vi "ep_EN50160 Basic Statistical Evaluation (1D).vi"(0 "data":dbl[](array[numeric]), 1 "evaluated data":enum16{"all data", "data without flag"}(ring), 5 "data flags":bool[](array[boolean]), 7 "EN50160 limits":T2={"upper limit"=110.0, "lower limit"=90.0, "required percentage to be in limits"=95.0}, 11 "error in (no error)":errorcluster) -> (4 "EN50160 result":T1, 10 "passed?":bool, 15 "error out":errorcluster)   [LabVIEW 2011, in "NI_EP_Power Quality.lvlib"]
uses:
  <vilib>/addons/Electrical Power/PQ/NI_EP_Power Quality.lvlib
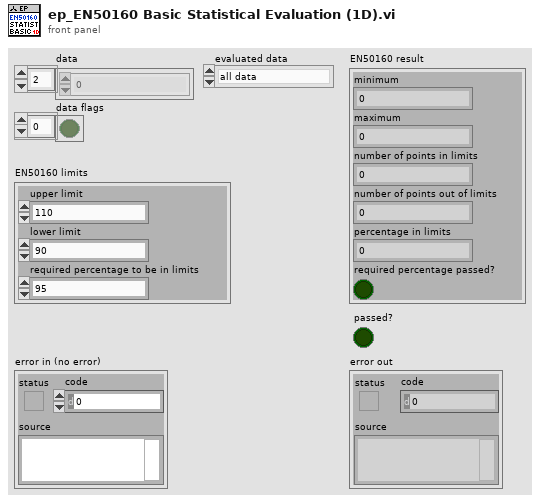
[diagram p1: front panel]
types:
  T1 = cluster{"minimum":dbl, "maximum":dbl, "number of points in limits":u32, "number of points out of limits":u32, "percentage in limits":dbl, "required percentage passed?":bool}
  T2 = cluster{"upper limit":dbl, "lower limit":dbl, "required percentage to be in limits":dbl}
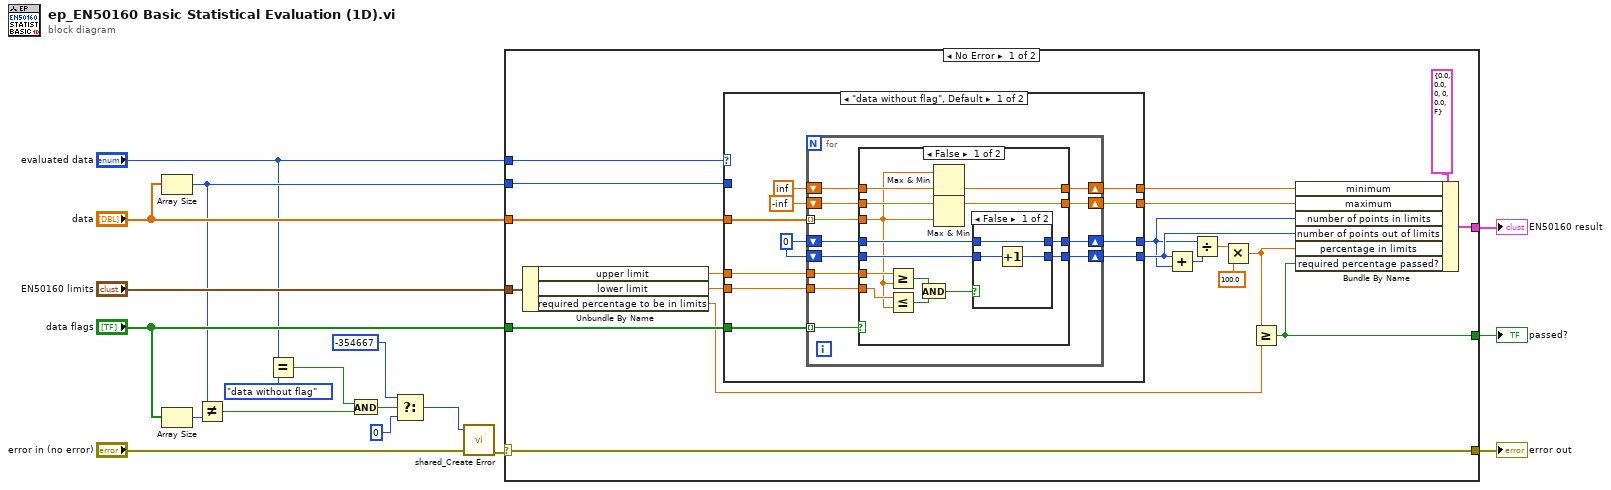
[diagram p0: block diagram]
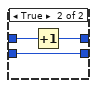
[diagram p2: hidden frame]
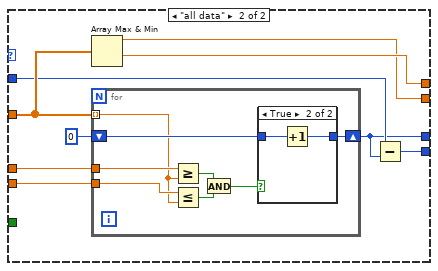
[diagram p4: hidden frame]
diagram:
  n1 = Array Size(array="data") -> (size(s)=w12:i32)
  n2 = Array Size(array="data flags") -> (size(s)=w16:i32)
  n3 = Not Equal?(x=w12, y=w16) -> (x != y?=w11:bool)
  n4 = Equal?(x="evaluated data", y=enum16{"all data", "data without flag"}."data without flag") -> (x = y?=w7:bool)
  n5 = And(x=w7, y=w11) -> (x .and. y?=w10:bool)
  n6 = Select(t=-354667 ("error code (0)"), s=w10, f=0 ("error code (0)")) -> (s? t:f=w1:i32)
  n7 = call <vilib>:"shared_Create Error.vi"("error in (no error)"="error in (no error)", "error code (0)"=w1) -> ("error out"=w2:errorcluster)  [unwired: 9 in]
  n8 = case shown="No Error" w2 {
    selector: w2 -> [w35 w106]
    tunnel: "evaluated data" -> [w33 _]
    tunnel: "data" -> [w34 _]
    tunnel: "data flags" -> [w38 _]
    tunnel: [w35 w106] -> w15
    tunnel: [w36 _] -> w14
    tunnel: "EN50160 limits" -> [w32 _]
    tunnel: w12 -> [w21 _]
    tunnel: [w19 _] -> w6
    frame No Error {
      n9 = Unbundle By Name(w32) -> ("upper limit"=w31:dbl, "lower limit"=w30:dbl, "required percentage to be in limits"=w22:dbl)
      n10 = case shown="\"data without flag\", Default" w33 {
        tunnel: w38 -> [w45 _]
        tunnel: w30 -> [w43 w92]
        tunnel: w34 -> [w49 w91]
        tunnel: w31 -> [w44 w93]
        tunnel: [w42 w90] -> w29
        tunnel: [w41 w89] -> w28
        tunnel: [w40 w87] -> w20
        tunnel: [w39 w86] -> w27
        tunnel: w21 -> [_ w88]
        frame "data without flag", Default {
          w48 = u32 0 ("number of points in limits")
          n11 = for {
            tunnel: w49 -> [w56] mode=indexing
            tunnel: w45 -> [w61] mode=indexing
            shift-right: [w58] -> w40
            shift-left: w48 -> [w57]
            tunnel: w44 -> [w60]
            tunnel: w43 -> [w59]
            shift-right: [w54] -> w39
            shift-left: w48 -> [w55]
            shift-right: [w53] -> w42
            shift-left: inf ("max value") -> [w52]
            shift-right: [w50] -> w41
            shift-left: -inf ("max value") -> [w51]
            n12 = case shown="False" w61 {
              tunnel: w60 -> [w75 _]
              tunnel: w59 -> [w74 _]
              tunnel: [w69 w85] -> w58
              tunnel: w57 -> [w70 w85]
              tunnel: w56 -> [w62 _]
              tunnel: w55 -> [w68 w84]
              tunnel: [w67 w84] -> w54
              tunnel: [w66 w83] -> w53
              tunnel: w52 -> [w64 w83]
              tunnel: w51 -> [w63 w82]
              tunnel: [w65 w82] -> w50
              frame False {
                n13 = Greater Or Equal?(x=w75, y=w62) -> (x >= y?=w73:bool)
                n14 = Less Or Equal?(x=w74, y=w62) -> (x <= y?=w72:bool)
                n15 = And(x=w73, y=w72) -> (x .and. y?=w71:bool)
                n16 = Max & Min(x=w62, y=w64) -> (min(x,y)=w66:dbl)  [unwired: 1 out]
                n17 = Max & Min(x=w63, y=w62) -> (max(x,y)=w65:dbl)  [unwired: 1 out]
                n18 = case shown="False" w71 {
                  tunnel: w70 -> [w76 w81]
                  tunnel: [w76 w80] -> w69
                  tunnel: w68 -> [w78 w79]
                  tunnel: [w77 w79] -> w67
                  frame False {
                    n19 = Increment(x=w78) -> (x+1=w77:u32)
                  }
                  frame True {
                    n20 = Increment(x=w81) -> (x+1=w80:u32)
                  }
                }
              }
              frame True {
                # "no evaluated data"
              }
            }
          }
        }
        frame "all data" {
          n21 = Array Max & Min(array=w91) -> (max value=w89:dbl, min value=w90:dbl)  [unwired: 2 out]
          n22 = for {
            tunnel: w91 -> [w98] mode=indexing
            shift-right: [w100] -> w87
            shift-left: u32 0 ("number of points in limits") -> [w99]
            tunnel: w93 -> [w102]
            tunnel: w92 -> [w101]
            n23 = Greater Or Equal?(x=w102, y=w98) -> (x >= y?=w97:bool)
            n24 = Less Or Equal?(x=w101, y=w98) -> (x <= y?=w96:bool)
            n25 = And(x=w97, y=w96) -> (x .and. y?=w95:bool)
            n26 = case shown="True" w95 {
              tunnel: w99 -> [w103 w105]
              tunnel: [w103 w104] -> w100
              frame False {
              }
              frame True {
                n27 = Increment(x=w105) -> (x+1=w104:u32)
              }
            }
          }
          n28 = Subtract(x=w88, y=w87) -> (x-y=w86:u32)
        }
      }
      n29 = Add(x=w27, y=w20) -> (x+y=w24:u32)
      n30 = Divide(x=w20, y=w24) -> (x/y=w26:dbl)
      n31 = Multiply(x=w26, y=100.0) -> (x*y=w23:dbl)
      n32 = Greater Or Equal?(x=w23, y=w22) -> (x >= y?=w19:bool)
      n33 = Bundle By Name(cluster=T1 {"minimum"=0.0, "maximum"=0.0, "number of points in limits"=0, "number of points out of limits"=0, "percentage in limits"=0.0, "required percentage passed?"=FALSE} ("EN50160 result"), "minimum"=w29, "maximum"=w28, "number of points in limits"=w20, "number of points out of limits"=w27, "percentage in limits"=w23, "required percentage passed?"=w19) -> (w36:T1)
    }
    frame Error {
    }
  }
  "EN50160 result" <- w14
  "error out" <- w15
  "passed?" <- w6
